vi "Find Potential CFTs.vi"(4 "dy":i32, 6 "dx":i32, 7 "Frame Number":i32, 8 "error in (no error)":errorcluster, 9 "ROI Height":i32, 10 "ROI Width":i32, 11 "Focused Image":T3) -> (0 "error out":errorcluster, 2 "Potential Tracks":T1[](array[typedef]) {"Line"."Start X" scale=0.0..1024.0; "Line"."End X" scale=0.0..1024.0}, 3 "Focused Image out":T3)   [LabVIEW 2013]
uses:
  <vilib>/vision/Image Controls.llb/IMAQ Image.ctl
  Scored Line.ctl
  <vilib>/vision/NI_Vision_Development_Module.lvlib
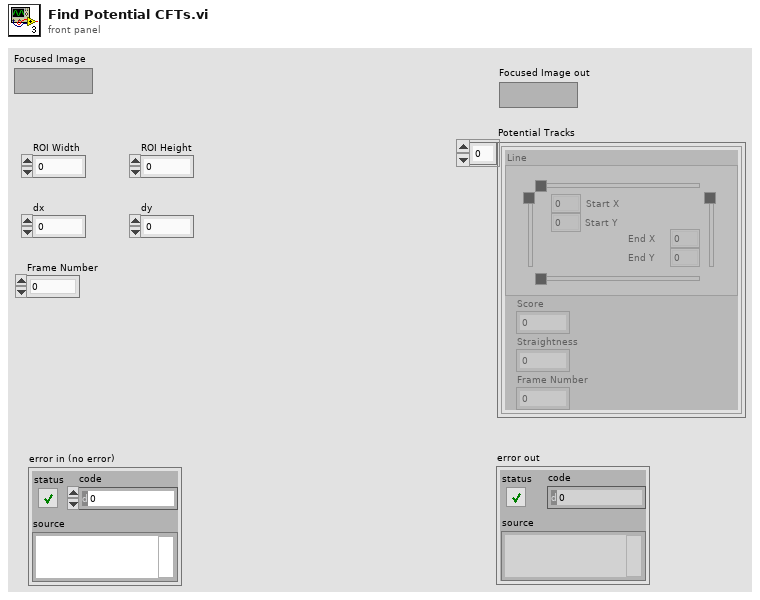
[diagram p1: front panel]
types:
  T1 = typedef "Scored Line.ctl" = cluster{"Line":T2, "Score":dbl, "Straightness":dbl, "Frame Number":i32}
  T2 = typedef "IMAQ Line" = cluster{"Start X":i32, "Start Y":i32, "End X":i32, "End Y":i32}
  T3 = typedef "IMAQ Image.ctl" = refnum<image>
  T4 = cluster{"Measurement Parameter":i32, "Range Lower Value":dbl, "Range Upper Value":dbl, "Range":bool, "Measurement Type":bool}[]
  T5 = typedef "IMAQ Rectangle" = cluster{"Left":i32, "Top":i32, "Right":i32, "Bottom":i32, "Rotation":dbl}
  T6 = enum32{"AutoM", "Close", "Dilate", "Erode", "Gradient", "Gradient out", "Gradient in", "Hit miss", "Open", "PClose", "POpen", "Thick", "Thin"}
  T7 = cluster{"Line":T2, "Score":dbl, "Straightness":dbl, "Frame Number":i32}
  T8 = typedef "ROI Descriptor" = cluster{"Global Rectangle":i32[], "Contours":cluster{"ID":enum32{"External", "Internal"}, "Type":u32, "Coordinates":i32[]}[]}
  T9 = cluster{"Point1 (Pixels)":cluster{"X":sgl, "Y":sgl}, "Point2 (Pixels)":cluster{"X":sgl, "Y":sgl}, "Point1 (Real-World)":cluster{"X":sgl, "Y":sgl}, "Point2 (Real-World)":cluster{"X":sgl, "Y":sgl}, "Angle (Pixel)":dbl, "Angle (Real-World)":dbl, "Score":dbl, "Straightness":dbl, "Average SNR (db)":dbl, "Calibration Valid":bool}[]
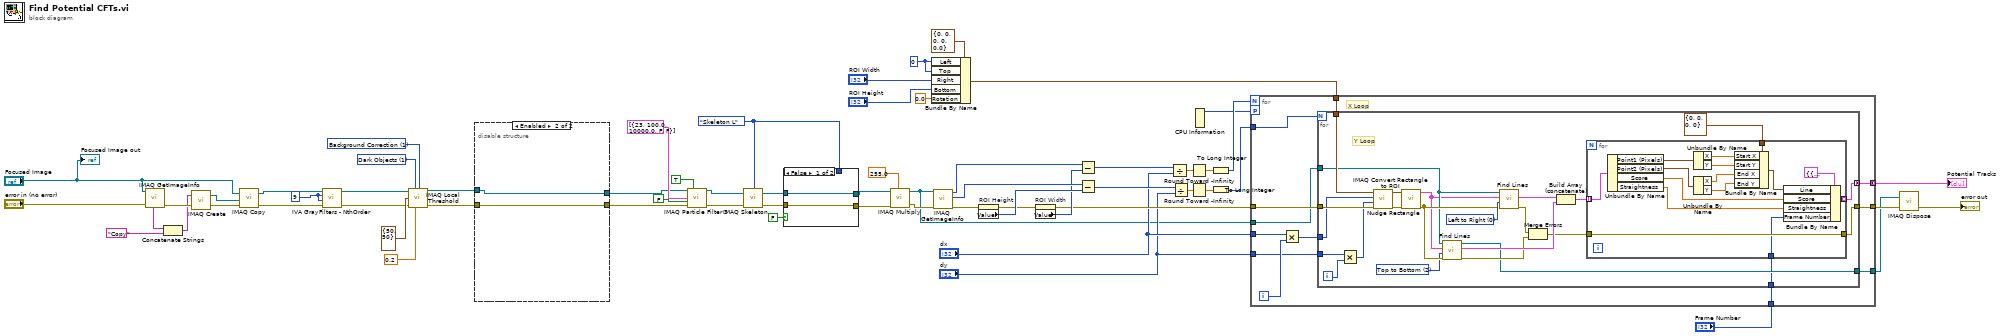
[diagram p0: block diagram]
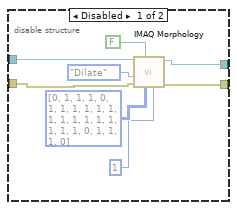
[diagram p2: hidden frame]
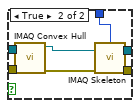
[diagram p3: hidden frame]
diagram:
  w10 = 9 ("Filter size X")
  w23 = enum32{"Skeleton L", "Skeleton M", "Skiz"}."Skeleton L" ("Mode")
  w36 = u32 1 items=["Bright Objects", "Dark Objects"] ("Look For (Bright Objects)")
  w37 = u32 1 items=["Niblack", "Background Correction"] ("Method (Niblack)")
  w63 = 0 ("Left")
  n1 = call "IMAQ GetImageInfo"("error in (no error)"="error in (no error)", "Image"="Focused Image") -> ("error out"=w40:errorcluster, "Image Name"=w39:string)  [unwired: 2 in, 6 out]
  n2 = Concatenate Strings(w39, "Copy" ("string")) -> (w38:string)
  n3 = call "IMAQ Create"("Image Name"=w38, "error in (no error)"=w40) -> ("New Image"=w14:T3, "error out"=w15:errorcluster)  [unwired: 3 in]
  n4 = call "IMAQ Copy"("error in (no error)"=w15, "Image Dst"=w14, "Image Src"="Focused Image") -> ("error out"=w11:errorcluster, "Image Dst Out"=w12:T3)  [unwired: 3 in]
  n5 = call <vilib>:"IVA GrayFilters - NthOrder.vi"("error in"=w11, "Filter size Y"=w10, "Filter size X"=w10, "Image In"=w12) -> ("error out"=w17:errorcluster, "Image Out"=w16:T3)  [unwired: 6 out]
  n6 = call "IMAQ Local Threshold"("Image Src"=w16, "Look For (Bright Objects)"=w36, "Method (Niblack)"=w37, "Window Size (32x32)"=cluster{"SizeX":i32, "SizeY":i32} {"SizeX"=50, "SizeY"=50} ("Kernel Size"), "error in (no error)"=w17, "Niblack Deviation Factor (0.2)"=0.2) -> ("Image Dst Out"=w4:T3, "error out"=w3:errorcluster)  [unwired: 2 in, 6 out]
  n7 = disable-structure shown="Enabled" {
    disable-tunnel: w4 -> [w72 w74]
    disable-tunnel: w3 -> [w71 w73]
    disable-tunnel: [w70 w74] -> w2
    disable-tunnel: [w69 w73] -> w1
    frame Disabled {
      n8 = call "IMAQ Morphology"("Number of iterations (1)"=1, "Structuring Element"=i32[][] [[0, 1, 1, 1, 0], [1, 1, 1, 1, 1], [1, 1, 1, 1, 1], [1, 1, 1, 1, 1], [0, 1, 1, 1, 0]], "Square/Hexa (Square)"=FALSE, "error in (no error)"=w71, "Operation"=T6."Dilate", "Image Src"=w72) -> ("error out"=w69:errorcluster, "Image Dst Out"=w70:T3)  [unwired: 1 in, 3 out]
    }
    frame Enabled {
    }
  }
  n9 = call "IMAQ Particle Filter 3"("Image Src"=w2, "Connectivity 4/8 (8)"=TRUE, "Selection Values"=T4 [{"Measurement Parameter"=23, "Range Lower Value"=100.0, "Range Upper Value"=10000.0, "Range"=FALSE, "Measurement Type"=FALSE}], "Keep/Remove Particles (F)"=FALSE ("Keep/Remove Particles"), "error in (no error)"=w1) -> ("Image Dst Out"=w6:T3, "error out"=w5:errorcluster)  [unwired: 4 in, 5 out]
  n10 = call "IMAQ Skeleton"("error in (no error)"=w5, "Image Src"=w6, "Mode"=w23) -> ("error out"=w24:errorcluster, "Image Dst Out"=w25:T3)  [unwired: 1 in, 2 out]
  n11 = case shown="False" FALSE {
    tunnel: w25 -> [w76 w83]
    tunnel: w24 -> [w75 w82]
    tunnel: w23 -> [_ w79]
    tunnel: [w76 w78] -> w22
    tunnel: [w75 w77] -> w21
    frame False {
    }
    frame True {
      n12 = call "IMAQ Convex Hull"("error in (no error)"=w82, "Image Src"=w83) -> ("error out"=w81:errorcluster, "Image Dst Out"=w80:T3)  [unwired: 8 in]
      n13 = call "IMAQ Skeleton"("error in (no error)"=w81, "Image Src"=w80, "Mode"=w79) -> ("error out"=w77:errorcluster, "Image Dst Out"=w78:T3)  [unwired: 1 in, 2 out]
    }
  }
  n14 = call "IMAQ Multiply"("Image Src A"=w22, "Constant"=sgl 255.0, "error in (no error)"=w21) -> ("Image Dst Out"=w29:T3, "error out"=w32:errorcluster)  [unwired: 4 in]
  n15 = Bundle By Name(cluster=T5 {"Left"=0, "Top"=0, "Right"=0, "Bottom"=0, "Rotation"=0.0} ("Rectangle"), "Left"=w63, "Top"=w63, "Right"="ROI Width", "Bottom"="ROI Height", "Rotation"=0.0) -> (w45:T5)
  n16 = call "IMAQ GetImageInfo"("error in (no error)"=w32, "Image"=w29) -> ("error out"=w59:errorcluster, "Y Resolution"=w57:i32, "X Resolution"=w55:i32)  [unwired: 2 in, 5 out]
  n17 = property on="ROI Height" class="DigNum (strict)"(error in=w59) -> (error out=w56:errorcluster, "Value"=w58:i32)  [unwired: 1 in, 1 out]
  n18 = property on="ROI Width" class="DigNum (strict)"(error in=w56) -> (error out=w44:errorcluster, "Value"=w54:i32)  [unwired: 1 in, 1 out]
  n19 = Subtract(x=w55, y=w54) -> (x-y=w53:i32)
  n20 = Subtract(x=w57, y=w58) -> (x-y=w52:i32)
  n21 = Divide(x=w53, y="dx") -> (x/y=w51:dbl)
  n22 = Divide(x=w52, y="dy") -> (x/y=w49:dbl)
  n23 = Round Toward -Infinity(1:w51) -> (0:w50:dbl)
  n24 = Round Toward -Infinity(1:w49) -> (0:w48:dbl)
  n25 = CPU Information() -> (4:w41:i32)  [unwired: 3 out]
  n26 = To Long Integer(number=w50) -> (32bit integer=w47:i32)
  n27 = To Long Integer(number=w48) -> (32bit integer=w46:i32)
  n28 = for {
    N: w47 -> [_]
    tunnel: w46 -> [w95]
    tunnel: w44 -> [w87]
    tunnel: w45 -> [w94]
    tunnel: "dx" -> [w93]
    tunnel: "dy" -> [w91]
    tunnel: [w89] -> w28
    tunnel: [w88] -> w18 mode=concatenating
    workers-P: w41 -> [_]
    tunnel: w29 -> [w86]
    tunnel: [w85] -> w27
    tunnel: "Frame Number" -> [w84]
    i -> [w92]
    # "X Loop"
    n29 = Multiply(x=w93, y=w92) -> (x*y=w90:i32)
    n30 = for {
      N: w95 -> [_]
      tunnel: w87 -> [w119]
      tunnel: w94 -> [w118]
      tunnel: w91 -> [w117]
      tunnel: w90 -> [w115]
      tunnel: w86 -> [w106]
      tunnel: [w109] -> w89
      tunnel: [w108] -> w88 mode=concatenating
      tunnel: [w97] -> w85
      tunnel: w84 -> [w96]
      i -> [w116]
      w104 = u32 2 items=["Left to Right", "Right to Left", "Top to Bottom", "Bottom to Top"] ("Search Direction")
      w111 = u32 0 items=["Left to Right", "Right to Left", "Top to Bottom", "Bottom to Top"] ("Search Direction")
      # "Y Loop"
      n31 = Multiply(x=w117, y=w116) -> (x*y=w114:i32)
      n32 = call "Nudge Rectangle.vi"("error in (no error)"=w119, "dy"=w114, "dx"=w115, "Rectangle"=w118) -> ("error out"=w113:errorcluster, "Nudged Rectangle"=w112:T5)  [unwired: 6 in]
      n33 = call "IMAQ Convert Rectangle to ROI"("error in (no error)"=w113, "Rectangle"=w112) -> ("error out"=w107:errorcluster, "ROI Descriptor"=w105:T8)  [unwired: 7 in]
      n34 = call "Find Lines.vi"("error in"=w107, "Search Direction"=w104, "ROI"=w105, "Image In"=w106) -> ("error out"=w98:errorcluster, "Straight Edges"=w101:T9, "Image Out"=w97:T3)  [unwired: 5 in]
      n35 = call "Find Lines.vi"("error in"=w107, "Search Direction"=w111, "ROI"=w105, "Image In"=w106) -> ("error out"=w100:errorcluster, "Straight Edges"=w103:T9)  [unwired: 5 in, 1 out]
      n36 = Merge Errors(w100, w98) -> (w99:errorcluster)
      n37 = Build Array (concatenate)(w103, w101) -> (w102:T9)
      n38 = for {
        tunnel: w99 -> [w123]
        tunnel: w102 -> [w134] mode=indexing
        tunnel: T2 {"Start X"=0, "Start Y"=0, "End X"=0, "End Y"=0} ("Line") -> [w131]
        tunnel: [w123] -> w109
        tunnel: [w122] -> w108 mode=indexing
        tunnel: w96 -> [w120]
        n39 = Unbundle By Name(w134) -> ("Point1 (Pixels)"=w133:cluster{"X":sgl, "Y":sgl}, "Point2 (Pixels)"=w132:cluster{"X":sgl, "Y":sgl}, "Score"=w125:dbl, "Straightness"=w124:dbl)
        n40 = Unbundle By Name(w133) -> ("X"=w130:sgl, "Y"=w129:sgl)
        n41 = Unbundle By Name(w132) -> ("X"=w128:sgl, "Y"=w127:sgl)
        n42 = Bundle By Name(cluster=w131, "Start X"=w130, "Start Y"=w129, "End X"=w128, "End Y"=w127) -> (w126:T2)
        n43 = Bundle By Name(cluster=T7 {"Line"={"Start X"=0, "Start Y"=0, "End X"=0, "End Y"=0}, "Score"=0.0, "Straightness"=0.0, "Frame Number"=0} ("Cluster"), "Line"=w126, "Score"=w125, "Straightness"=w124, "Frame Number"=w120) -> (w122:T7)
      }
    }
  }
  "Potential Tracks" <- w18
  n44 = call "IMAQ Dispose"("Image"=w27, "error in (no error)"=w28) -> ("error out"=→"error out":errorcluster)  [unwired: 4 in]
  "Focused Image out" <- "Focused Image"
